vi "Global Log To String.vi"(10 "Log":T1) -> (3 "String":string)   [LabVIEW 2014, in "JKI State Machine++.lvlib"]
uses:
  JKI State Machine++.lvlib
  _Support/Typedef/_JKISM_GlobalLog_MSG_TYPE.ctl
  _Support/Typedef/_JKISM_GlobalLog_MSG.ctl
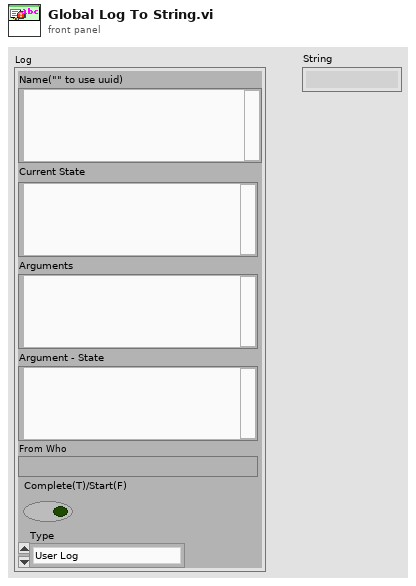
[diagram p1: front panel]
types:
  T1 = typedef "JKI State Machine++.lvlib/_JKISM_GlobalLog_MSG.ctl" = cluster{"Name(\"\" to use uuid)":string, "Current State":string, "Arguments":string, "Argument - State":string, "From Who":string, "Complete(T)/Start(F)":bool, "Type":T2}
  T2 = typedef "JKI State Machine++.lvlib/_JKISM_GlobalLog_MSG_TYPE.ctl" = enum16{"User Log", "State Change", "Status", "Interrupt", "Register", "Unregister"}
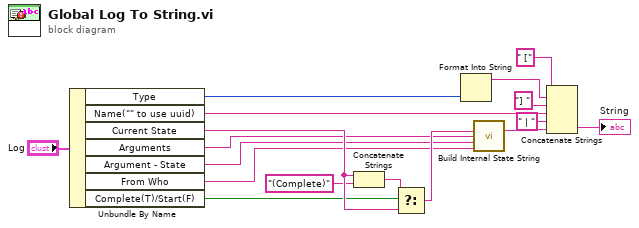
[diagram p0: block diagram]
diagram:
  n1 = Unbundle By Name("Log") -> ("Type"=w16:T2, "Name(\"\" to use uuid)"=w3:string, "Current State"=w12:string, "Arguments"=w4:string, "Argument - State"=w5:string, "From Who"=w6:string, "Complete(T)/Start(F)"=w10:bool)
  n2 = Concatenate Strings(w12, "(Complete)" ("string")) -> (w11:string)
  n3 = Select(t=w11, s=w10, f=w12) -> (s? t:f=w13:string)
  n4 = Format Into String(w16) -> (resulting string=w17:string)  [unwired: 3 in, 1 out]
  n5 = call "Build Internal State String.vi"("State"=w13, "Arguments (\"\")"=w4, "Arg-State (\"\")"=w5, "Source (\"\")"=w6) -> ("State with Arguments"=w8:string)  [unwired: 11 in]
  n6 = Concatenate Strings(" [" ("string"), w17, "] " ("string"), w3, " | " ("string"), w8) -> (→"String":string)
